vi "SA Cond - t0; Time Align Signals.vi"(0 "Signal IN":waveform(dbl)[](array[waveform]), 5 "error in (no error)":errorcluster, 6 "Anotate Signal Name":bool=TRUE) -> (14 "Signal OUT":waveform(dbl)[](array[waveform]), 19 "error out":errorcluster)   [LabVIEW 2020, in "GSwFormDSP.lvclass"]
uses:
  GSwFormDSP.lvclass
  <userlib>/_OpenG.lib/array/array.llb/Remove Duplicates from 1D Array (String)__ogtk.vi
  functions/Attribute List.ctl
  functions/Attribute Options.ctl
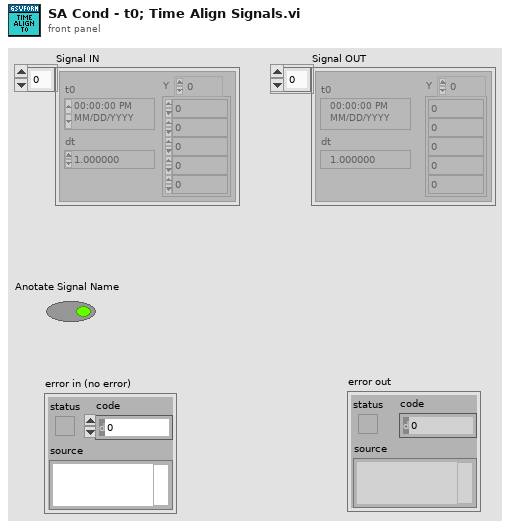
[diagram p1: front panel]
types:
  T1 = typedef "GSwFormDSP.lvclass/Attribute List.ctl" = string
  T2 = typedef "GSwFormDSP.lvclass/Attribute Options.ctl" = enum16{"Append to Attribute using \"( )\"", "Replace Attribute Value"}
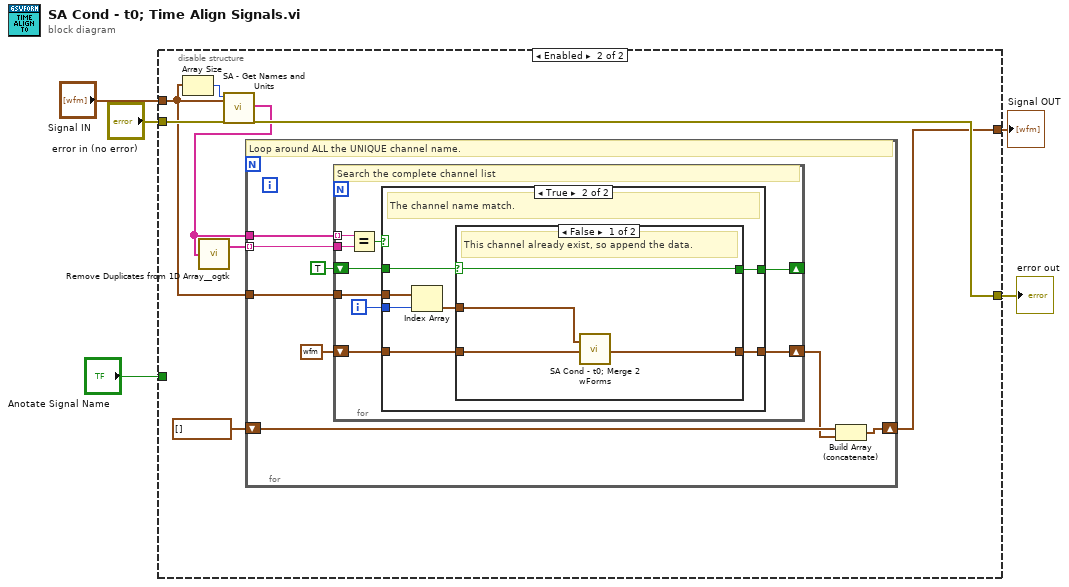
[diagram p0: block diagram]
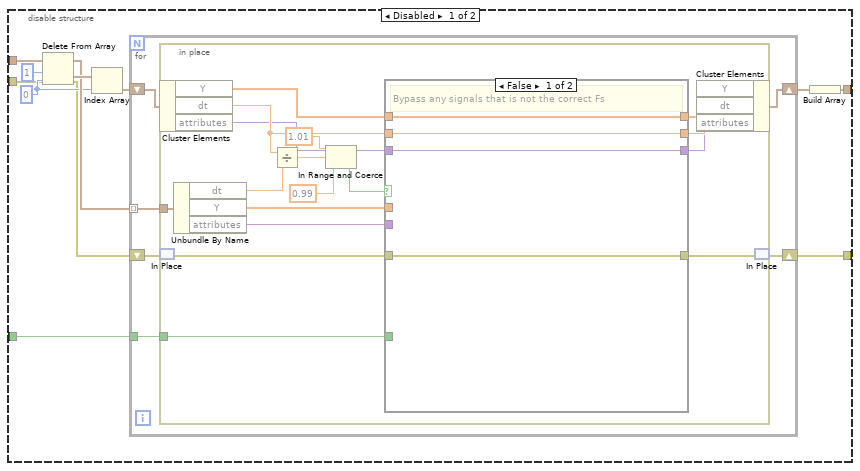
[diagram p2: hidden frame]
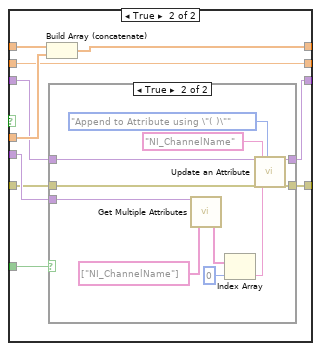
[diagram p3: hidden frame]
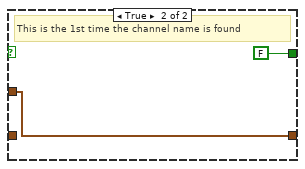
[diagram p6: hidden frame]
diagram:
  n1 = disable-structure shown="Enabled" {
    disable-tunnel: [w16 w67] -> w5
    disable-tunnel: "Signal IN" -> [w15 w69]
    disable-tunnel: "Anotate Signal Name" -> [w8 _]
    disable-tunnel: "error in (no error)" -> [w7 w73]
    disable-tunnel: [w6 w72] -> w1
    frame Disabled {
      w10 = 0 ("index")
      n2 = Delete From Array(array=w15, length=1, index=w10) -> (deleted portion=w13:waveform(dbl)[], array with subset deleted=w11:waveform(dbl)[])
      n3 = Index Array(array=w13, index=w10) -> (element=w12:waveform(dbl))
      n4 = for {
        shift-right: [w20] -> w9
        shift-left: w12 -> [w22]
        tunnel: w11 -> [w21] mode=indexing
        tunnel: w8 -> [w19]
        shift-right: [w17] -> w6
        shift-left: w7 -> [w18]
        n5 = in-place {
          in-place-border: w21 -> [w38]
          in-place-border: w19 -> [w29]
          n6 = in-place-cluster #1(w22) -> ("Y"=w39:dbl[], "dt"=w33:dbl, "attributes"=w32:variant)
          n7 = in-place-match #2(w18) -> (w28:errorcluster)
          n8 = Unbundle By Name(w38) -> ("dt"=w37:dbl, "Y"=w36:dbl[], "attributes"=w30:variant)
          n9 = Divide(x=w33, y=w37) -> (x/y=w26:dbl)
          n10 = In Range and Coerce(upper limit=1.01, x=w26, lower limit=0.99) -> (In Range?=w25:bool)  [unwired: 1 out]
          n11 = case shown="False" w25 {
            tunnel: w39 -> [w43 w53]
            tunnel: w36 -> [_ w52]
            tunnel: [w43 w51] -> w35
            tunnel: [w42 w50] -> w34
            tunnel: w33 -> [w42 w50]
            tunnel: w32 -> [w41 w49]
            tunnel: [w41 w47] -> w31
            tunnel: w30 -> [_ w48]
            tunnel: w29 -> [_ w46]
            tunnel: w28 -> [w40 w45]
            tunnel: [w40 w44] -> w27
            frame False {
              # "Bypass any signals that is not the correct Fs"
            }
            frame True {
              n12 = Build Array (concatenate)(w53, w52) -> (w51:dbl[])
              n13 = case shown="True" w46 {
                tunnel: w49 -> [w55 w66]
                tunnel: [w55 w65] -> w47
                tunnel: w48 -> [_ w64]
                tunnel: w45 -> [w54 w57]
                tunnel: [w54 w56] -> w44
                frame False {
                }
                frame True {
                  n14 = call "Get Multiple Attributes.vi"("Attributes IN"=w64, "Attribute List"=T1[] ["NI_ChannelName"]) -> ("Values"=w62:string[])  [unwired: 16 in, 1 out]
                  n15 = Index Array(array=w62, index=0) -> (element=w60:string)
                  n16 = call "Update an Attribute.vi"("attributes in"=w66, "error in (no error)"=w57, "Attribute List"=T1 "NI_ChannelName", "Attribute Value"=w60, "Attribute Option"=Attribute_Options."Append to Attribute using \"( )\"") -> ("attributes out"=w65:variant, "error out"=w56:errorcluster)  [unwired: 13 in]
                }
              }
            }
          }
          n17 = in-place-cluster #1("Y"=w35, "dt"=w34, "attributes"=w31) -> (w20:waveform(dbl))
          n18 = in-place-match #2(w27) -> (w17:errorcluster)
        }
      }
      n19 = Build Array(w9) -> (w16:waveform(dbl)[])
    }
    frame Enabled {
      n20 = Array Size(array=w69) -> (size(s)=w74:i32)
      n21 = call "SA - Get Names and Units.vi"("Nb Signals"=w74, "Signal IN"=w69, "error in (no error)"=w73) -> ("Signal Names"=w70:string[], "error out"=w72:errorcluster)  [unwired: 12 in, 3 out]
      n22 = call-poly <userlib>:"Remove Duplicates from 1D Array__ogtk.vi"("Input Array"=w70) -> ("Output Array"=w71:string[])  [unwired: 1 out]
      n23 = for {
        tunnel: w71 -> [w81] mode=indexing
        tunnel: w70 -> [w82]
        shift-right: [w77] -> w67
        shift-left: waveform(dbl)[] [] ("Signal IN") -> [w78]
        tunnel: w69 -> [w80]
        # "Loop around ALL the UNIQUE channel name."
        n24 = for {
          tunnel: w81 -> [w91]
          tunnel: w82 -> [w90] mode=indexing
          tunnel: w80 -> [w87]
          shift-right: [w85] -> _
          shift-left: TRUE -> [w86]
          shift-right: [w84] -> w76
          shift-left: waveform(dbl) {"t0"=timestamp(0 s since 1904-01-01), "dt"=1.0, "Y"=[]} ("Waveform") -> [w83]
          i -> [w88]
          # "Search the complete channel list"
          n25 = Equal?(x=w90, y=w91) -> (x = y?=w89:bool)
          n26 = case shown="True" w89 {
            tunnel: w88 -> [_ w100]
            tunnel: w87 -> [_ w99]
            tunnel: w86 -> [w93 w98]
            tunnel: [w93 w97] -> w85
            tunnel: [w92 w96] -> w84
            tunnel: w83 -> [w92 w94]
            frame False {
              # "Channel name does NOT match, do nothing."
            }
            frame True {
              # "The channel name match."
              n27 = Index Array(array=w99, index=w100) -> (element=w95:waveform(dbl))
              n28 = case shown="False" w98 {
                selector: w98 -> [w104 _]
                tunnel: [w104 FALSE] -> w97
                tunnel: [w102 w105] -> w96
                tunnel: w95 -> [w101 w105]
                tunnel: w94 -> [w103 _]
                frame False {
                  # "This channel already exist, so append the data."
                  n29 = call "SA Cond - t0; Merge 2 wForms.vi"("Waveform IN 2"=w101, "Waveform IN 1"=w103) -> ("Merged Waveform"=w102:waveform(dbl))  [unwired: 17 in]
                }
                frame True {
                  # "This is the 1st time the channel name is found"
                }
              }
            }
          }
        }
        n30 = Build Array (concatenate)(w78, w76) -> (w77:waveform(dbl)[])
      }
    }
  }
  "Signal OUT" <- w5
  "error out" <- w1
